vi "Volt_to_Angle.vi"(11 "Dynamic Data Type":dbl) -> (3 "Angle":dbl[](array[numeric]))   [LabVIEW 2022 SP3]
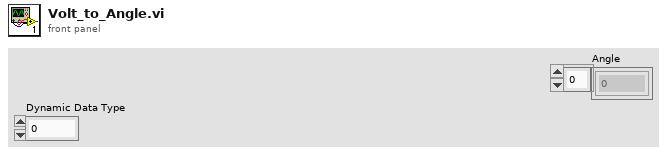
[diagram p1: front panel]
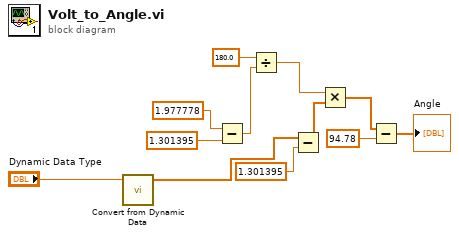
[diagram p0: block diagram]
diagram:
  n1 = call "Convert from Dynamic Data"("Dynamic Data Type"="Dynamic Data Type") -> ("Array"=w2:dbl[])  [unwired: 3 in]
  n2 = Subtract(x=1.977778, y=1.301395) -> (x-y=w9:dbl)
  n3 = Divide(x=180.0, y=w9) -> (x/y=w8:dbl)
  n4 = Subtract(x=w2, y=1.301395) -> (x-y=w6:dbl[])
  n5 = Multiply(x=w8, y=w6) -> (x*y=w5:dbl[])
  n6 = Subtract(x=w5, y=94.78) -> (x-y=→"Angle":dbl[])
